vi "Read JSON Config.vi"(8 "error in (no error)":errorcluster, 10 "JSON Config":string, 11 "Const_DBL in":refnum<class "Const_DBL.lvclass">) -> (0 "error out":errorcluster, 3 "Const_DBL out":refnum<class "Const_DBL.lvclass">)   [LabVIEW 2021, in "Const_DBL.lvclass"]
uses:
  Const_DBL.lvclass
  C:/Program Files (x86)/National Instruments/LabVIEW 2021/vi.lib/TSA/Abstract Data Classes/Abs_Types/Type/Abs_Type.lvclass
  Const_DBL.lvclass/Const_DBL.ctl
  68bfc6fe-4910-4c76-bc57-099680d7e0a2.vi
  <vilib>/JDP Science/JSONtext/Find Item.vi
  <vilib>/JDP Science/JSONtext/Next JSON Value.vi
  <vilib>/JDP Science/JSONtext/String Subset.vi
  <vilib>/JDP Science/JSONtext/Parsing/Advance past next JSON Value (inlined COPY).vi
  <vilib>/JDP Science/JSONtext/Parsing/Advance past whitespace.vi
  <vilib>/JDP Science/JSONtext/Parsing/Advance past String.vi
  <vilib>/JDP Science/JSONtext/Parsing/Advance past Number.vi
  <vilib>/JDP Science/JSONtext/Parsing/Advance past Line Ending.vi
  <vilib>/Utility/LVClass/Get LV Class Name.vi
  <vilib>/JDP Science/JSONtext/Parsing/Parse Full Path or Item Name.vi
  <vilib>/JDP Science/JSONtext/Parsing/Advance past Array.vi
  <vilib>/JDP Science/JSONtext/Parsing/Advance past Object.vi
  <vilib>/JDP Science/JSONtext/support/Error Cluster From Code.vi
  <vilib>/JDP Science/JSONtext/Offset/Find Item Locations by Path.vi
  <vilib>/JDP Science/JSONtext/JSON text to Variant.vi
  <vilib>/JDP Science/JSONtext/LVClass Serializer/JSONtext LVClass Serializer.lvclass
  Abs_Types/Double Float/Abs_Double Float.lvclass
  Abs_Types/Type/Abs_Type.lvclass
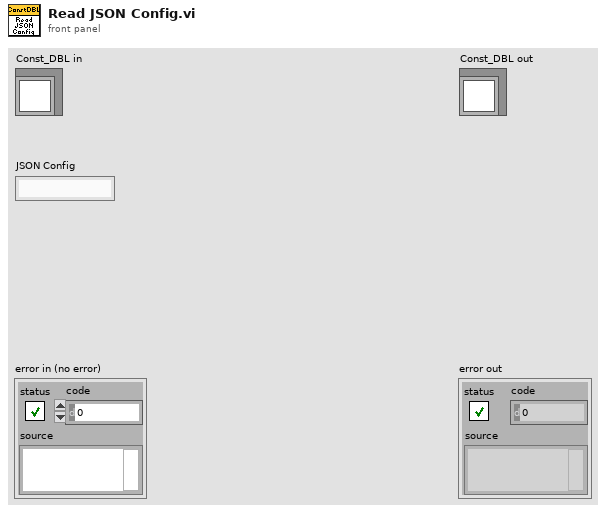
[diagram p1: front panel]
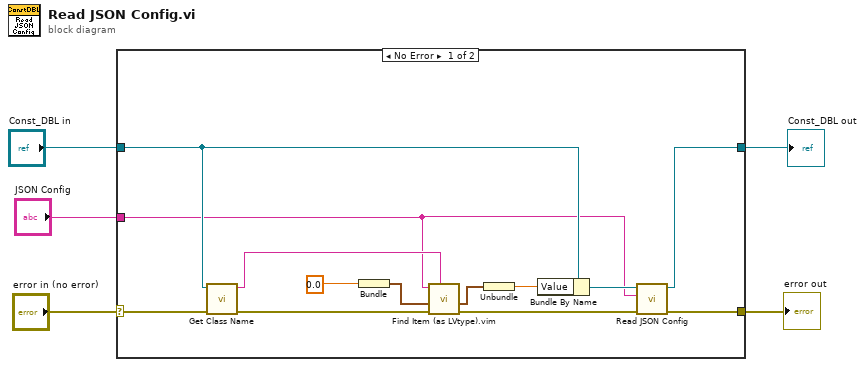
[diagram p0: block diagram]
diagram:
  n1 = case shown="No Error" "error in (no error)" {
    selector: "error in (no error)" -> [w12 w19]
    tunnel: [w18 w19] -> w2
    tunnel: [w17 w20] -> w1
    tunnel: "JSON Config" -> [w7 _]
    tunnel: "Const_DBL in" -> [w9 w20]
    frame No Error {
      n2 = call "Get Class Name.vi"("error in (no error)"=w12, "Abs_Type in"=w9) -> ("error out"=w10:errorcluster, "class name"=w11:string)  [unwired: 8 in]
      n3 = Bundle("Value"=0.0) -> (w14:cluster{"Value":dbl})  [unwired: 1 in]
      n4 = call "Find Item (as LVtype).vim"("$Path or Item Name"=w11, "error in (no error)"=w10, "Data Type and Default Value"=w14, "JSON"=w7) -> ("error out"=w13:errorcluster, "Data"=w15:cluster{"Value":dbl})  [unwired: 4 in, 2 out]
      n5 = Unbundle(w15) -> ("Value"=w16:dbl)
      n6 = Bundle By Name(cluster=w9, "Value"=w16) -> (w8:refnum<class "Const_DBL.lvclass">)
      n7 = call-parent "Read JSON Config.vi"("error in (no error)"=w13, "JSON Config"=w7, "Abs_Type in"=w8) -> ("error out"=w18:errorcluster, "Abs_Type out"=w17:refnum<class "Const_DBL.lvclass">)  [unwired: 7 in]
    }
    frame Error {
    }
  }
  "error out" <- w2
  "Const_DBL out" <- w1
